vi "Pre Launch Init.vi"(11 "Command Handler in":refnum<class "Command Handler.lvclass">) -> (0 "error out":errorcluster, 3 "Command Handler out":refnum<class "Command Handler.lvclass">)   [LabVIEW 2017, in "Command Handler.lvlib" / "Command Handler.lvclass"]
doc: "(<B>Filename</B>: Actor Framework.lvlib:Actor.lvclass:Pre Launch Init.vi)\n\nDefines behavior that occurs after the Launch Nested Actor method is invoked but before the actor's Actor Core method begins running.\n\nBy default, this method does nothing. A descendant class may override it to define behavior."
uses:
  Command Handler.lvclass
  Command Parents/Command.lvclass
  Type Defs/Command Handler Data.ctl
  Command Handler.lvclass/Command Handler.ctl
  <vilib>/ActorFramework/Actor/Actor.lvclass
  Command Handler.lvlib
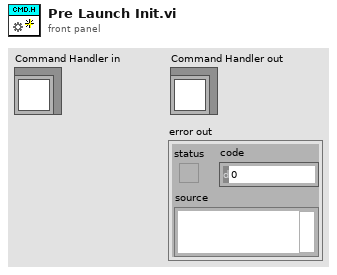
[diagram p1: front panel]
types:
  T1 = typedef "Command Handler.lvlib/Command Handler.lvclass/Command Handler Data.ctl" = cluster{"Commands Loaded":i32, "Loaded Command Names":string[], "Commands Completed":i32, "Completed Command Names":string[]}
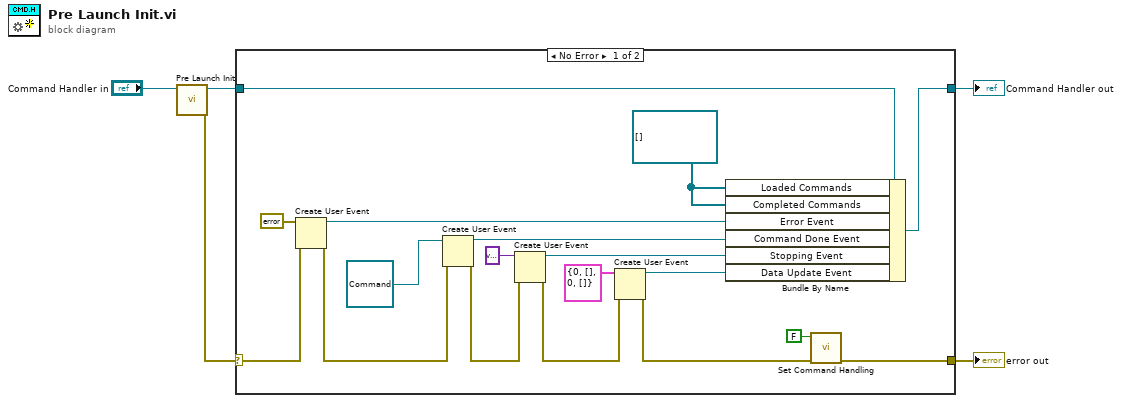
[diagram p0: block diagram]
diagram:
  n1 = call-parent "Pre Launch Init.vi"("Actor in"="Command Handler in") -> ("error out"=w1:errorcluster, "Actor out"=w4:refnum<class "Command Handler.lvclass">)  [unwired: 9 in]
  n2 = case shown="No Error" w1 {
    selector: w1 -> [w10 w24]
    tunnel: w4 -> [w21 w25]
    tunnel: [w20 w25] -> w3
    tunnel: [w6 w24] -> w2
    frame No Error {
      w14 = refnum<class "Command.lvclass">[] [] ("Completed Commands")
      n3 = Create User Event(user event datatype=errorcluster {"status"=FALSE, "code"=0, "source"=""} ("error in (no error)"), error in=w10) -> (user event=w23:refnum<user-event>, error out=w18:errorcluster)
      n4 = Create User Event(user event datatype=refnum<class "Command.lvclass"> refnum ("Command Library.lvlib:Command.lvclass"), error in=w18) -> (user event=w19:refnum<user-event>, error out=w15:errorcluster)
      n5 = Create User Event(user event datatype=variant ("error in (no error)"), error in=w15) -> (user event=w17:refnum<user-event>, error out=w11:errorcluster)
      n6 = Create User Event(user event datatype=T1 {"Commands Loaded"=0, "Loaded Command Names"=[], "Commands Completed"=0, "Completed Command Names"=[]} ("Sequencer Data"), error in=w11) -> (user event=w12:refnum<user-event>, error out=w7:errorcluster)
      n7 = Bundle By Name(cluster=w21, "Loaded Commands"=w14, "Completed Commands"=w14, "Error Event"=w23, "Command Done Event"=w19, "Stopping Event"=w17, "Data Update Event"=w12) -> (w20:refnum<class "Command Handler.lvclass">)
      n8 = call "Set Command Handling.vi"("error in (no error)"=w7, "Disable Command Handling"=FALSE ("Command Handling Stopped")) -> ("error out"=w6:errorcluster)  [unwired: 9 in]
    }
    frame Error {
    }
  }
  "error out" <- w2
  "Command Handler out" <- w3
